vi "Write Radius (px).vi"(8 "error in (no error)":errorcluster, 10 "Radius (px)":u16, 11 "Geometric Figure in":refnum<class "UI Object.lvclass">) -> (0 "error out":errorcluster, 3 "Geometric Figure out":refnum<class "UI Object.lvclass">)   [LabVIEW 2016]
uses:
  UI Object.lvclass
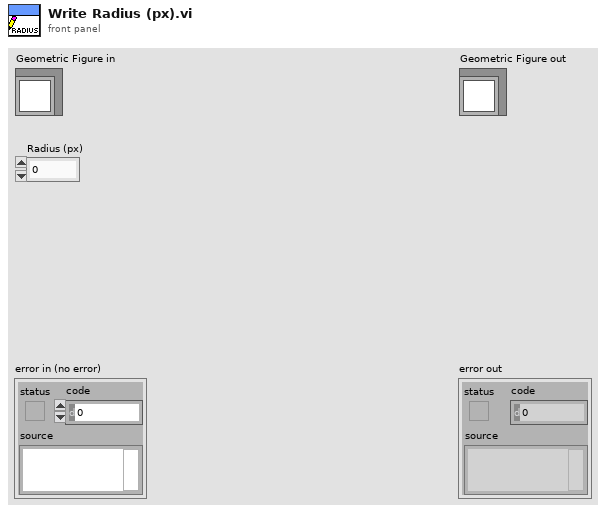
[diagram p1: front panel]
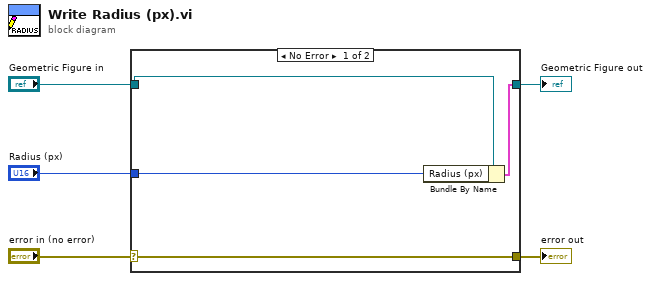
[diagram p0: block diagram]
diagram:
  n1 = case shown="No Error" "error in (no error)" {
    selector: "error in (no error)" -> [w9 w10]
    tunnel: [w9 w10] -> w4
    tunnel: [w7 w11] -> w2
    tunnel: "Geometric Figure in" -> [w8 w11]
    tunnel: "Radius (px)" -> [w6 _]
    frame No Error {
      n2 = Bundle By Name(cluster=w8, "Radius (px)"=w6) -> (w7:cluster{})
    }
    frame Error {
    }
  }
  "error out" <- w4
  "Geometric Figure out" <- w2
